vi "Timeout.vi"(8 "error in (no error)":errorcluster, 11 "SwipeMenu in":refnum<class "SwipeMenu.lvclass">) -> (0 "error out":errorcluster, 3 "SwipeMenu out":refnum<class "SwipeMenu.lvclass">)   [LabVIEW 2019, in "SwipeMenu.lvclass"]
uses:
  SwipeMenu.lvclass
  SwipeMenu.lvclass/SwipeMenu.ctl
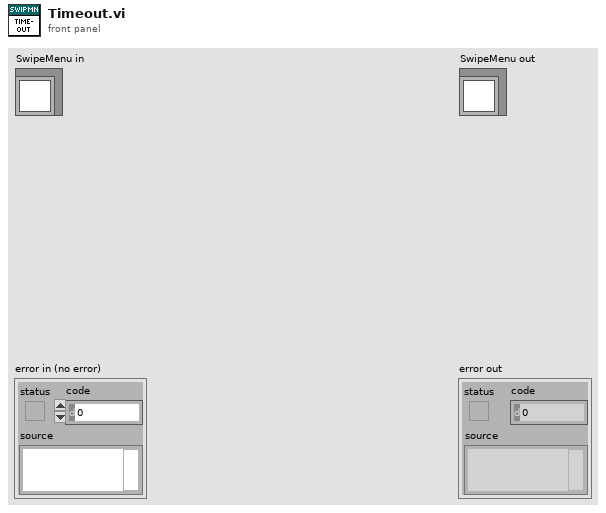
[diagram p1: front panel]
types:
  T1 = typedef "SwipeMenu.lvclass/State Data.ctl" = cluster{"State":enum16{"Idle", "Mouse Nav", "Slowdown", "Button Nav"}, "Timeout":i32, "Time":timestamp, "Position":i32, "Scroll Position":i16, "Rate":dbl, "Direction":enum16{"Left", "Right"}}
  T2 = enum16{"Idle", "Mouse Nav", "Slowdown", "Button Nav"}
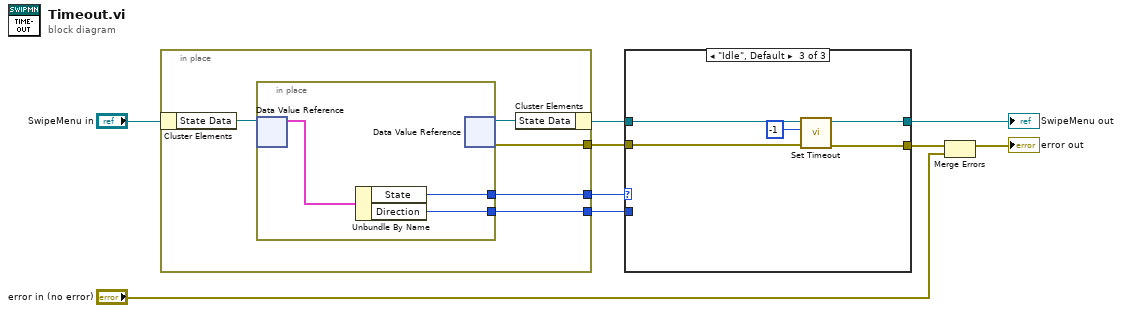
[diagram p0: block diagram]
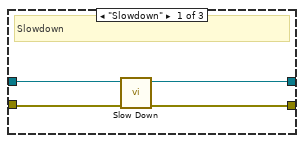
[diagram p2: hidden frame]
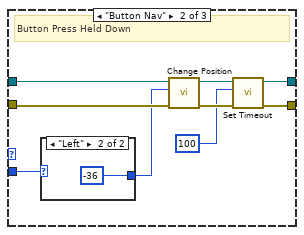
[diagram p3: hidden frame]
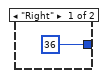
[diagram p4: hidden frame]
diagram:
  n1 = in-place {
    in-place-border: [w12] -> w6
    in-place-border: [w11] -> w5
    in-place-border: [w10] -> w1
    n2 = in-place-cluster #1("SwipeMenu in") -> ("State Data"=w14:refnum<data-value>)
    n3 = in-place {
      in-place-border: [w16] -> w12
      in-place-border: [w15] -> w10
      n4 = in-place-dvr #2(w14) -> (w17:T1)  [unwired: 1 out]
      n5 = Unbundle By Name(w17) -> ("State"=w15:T2, "Direction"=w16:enum16{"Left", "Right"})
      n6 = in-place-dvr #2() -> (w13:refnum<data-value>, w11:errorcluster)  [unwired: 1 in]
    }
    n7 = in-place-cluster #1("State Data"=w13) -> (w8:refnum<class "SwipeMenu.lvclass">)
  }
  n8 = case shown="\"Idle\", Default" w1 {
    tunnel: w8 -> [w21 w30 w37]
    tunnel: [w20 w25 w34] -> w7
    tunnel: w6 -> [_ w27 _]
    tunnel: w5 -> [w19 w29 w36]
    tunnel: [w18 w22 w33] -> w4
    frame "Slowdown" {
      # "Slowdown"
      n9 = call "Slow Down.vi"("error in (no error)"=w19, "SwipeMenu in"=w21) -> ("error out"=w18:errorcluster, "SwipeMenu out"=w20:refnum<class "SwipeMenu.lvclass">)  [unwired: 8 in]
    }
    frame "Button Nav" {
      # "Button Press Held Down"
      n10 = case shown="\"Left\"" w27 {
        tunnel: [i16 36 ("Change Position") i16 -36 ("Change Position")] -> w28
        frame "Right" {
        }
        frame "Left" {
        }
      }
      n11 = call "Change Position.vi"("error in (no error)"=w29, "Change Position"=w28, "SwipeMenu in"=w30) -> ("error out"=w24:errorcluster, "SwipeMenu out"=w26:refnum<class "SwipeMenu.lvclass">)  [unwired: 6 in, 1 out]
      n12 = call "Set Timeout.vi"("error in (no error)"=w24, "Timeout"=100, "SwipeMenu in"=w26) -> ("error out"=w22:errorcluster, "SwipeMenu out"=w25:refnum<class "SwipeMenu.lvclass">)  [unwired: 7 in]
    }
    frame "Idle", Default {
      n13 = call "Set Timeout.vi"("error in (no error)"=w36, "Timeout"=-1, "SwipeMenu in"=w37) -> ("error out"=w33:errorcluster, "SwipeMenu out"=w34:refnum<class "SwipeMenu.lvclass">)  [unwired: 7 in]
    }
  }
  "SwipeMenu out" <- w7
  n14 = Merge Errors(w4, "error in (no error)") -> (→"error out":errorcluster)
